vi "Processing_description.vi"(7 "type":enum16{"int", "float"}(ring)=enum."float", 8 "error in":errorcluster, 11 "Ответ устройства":string) -> (0 "error out":errorcluster, 2 "Param":T1, 4 "Тип/версия устройства":string, 6 "appended array":string[](array[string]))   [LabVIEW 2017, in "LV_Unicorn.lvlib"]
uses:
  LV_Unicorn.lvlib
  Control/unicorn_DescriptParam.ctl
panel:
  out "length":i32
  out "substring before match":string
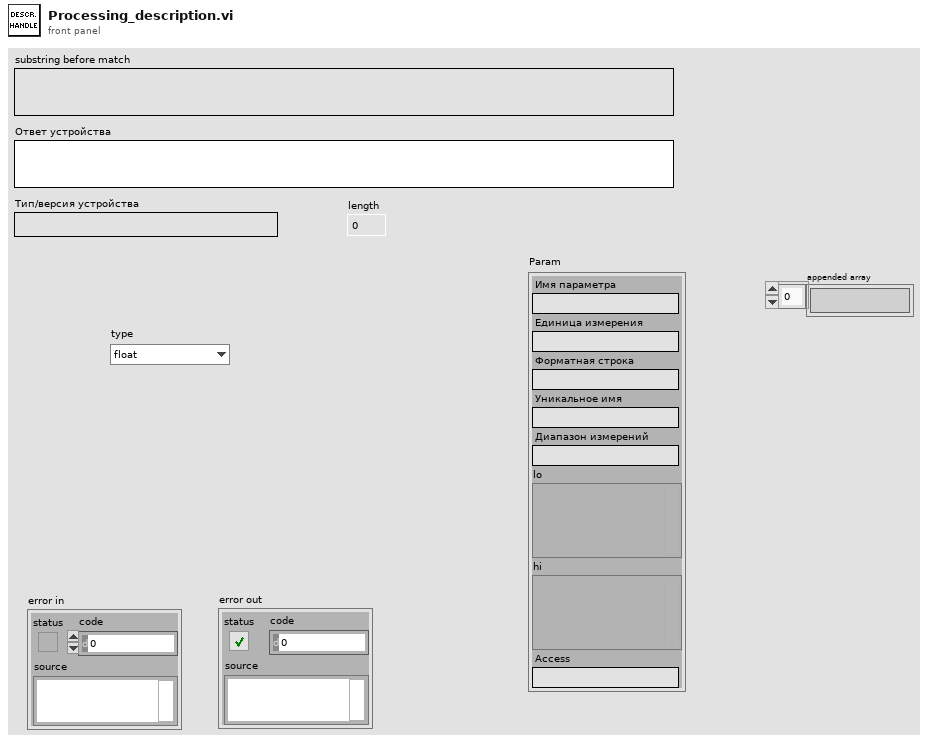
[diagram p1: front panel]
types:
  T1 = typedef "unicorn_DescriptParam.ctl" = cluster{"Имя параметра":string, "Единица измерения":string, "Форматная строка ":string, "Уникальное имя":string, "Диапазон измерений":string, "lo":variant, "hi":variant, "Access":string}
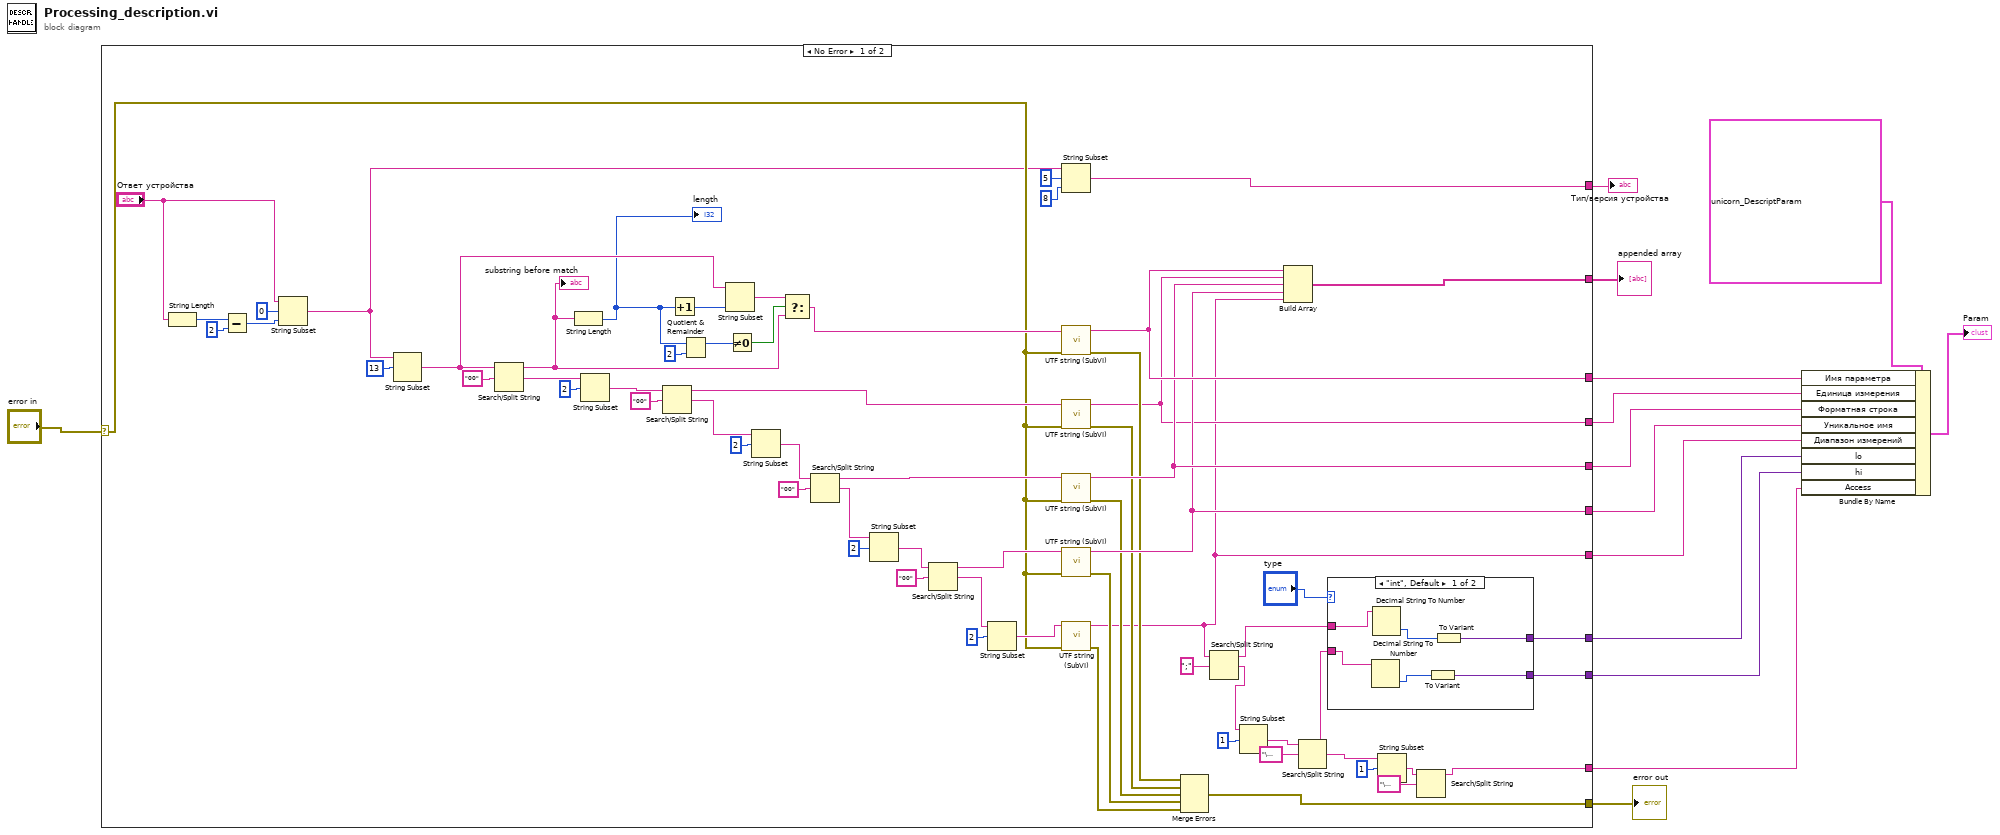
[diagram p0: block diagram]
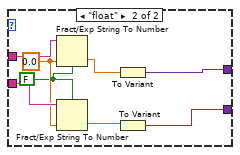
[diagram p2: hidden frame]
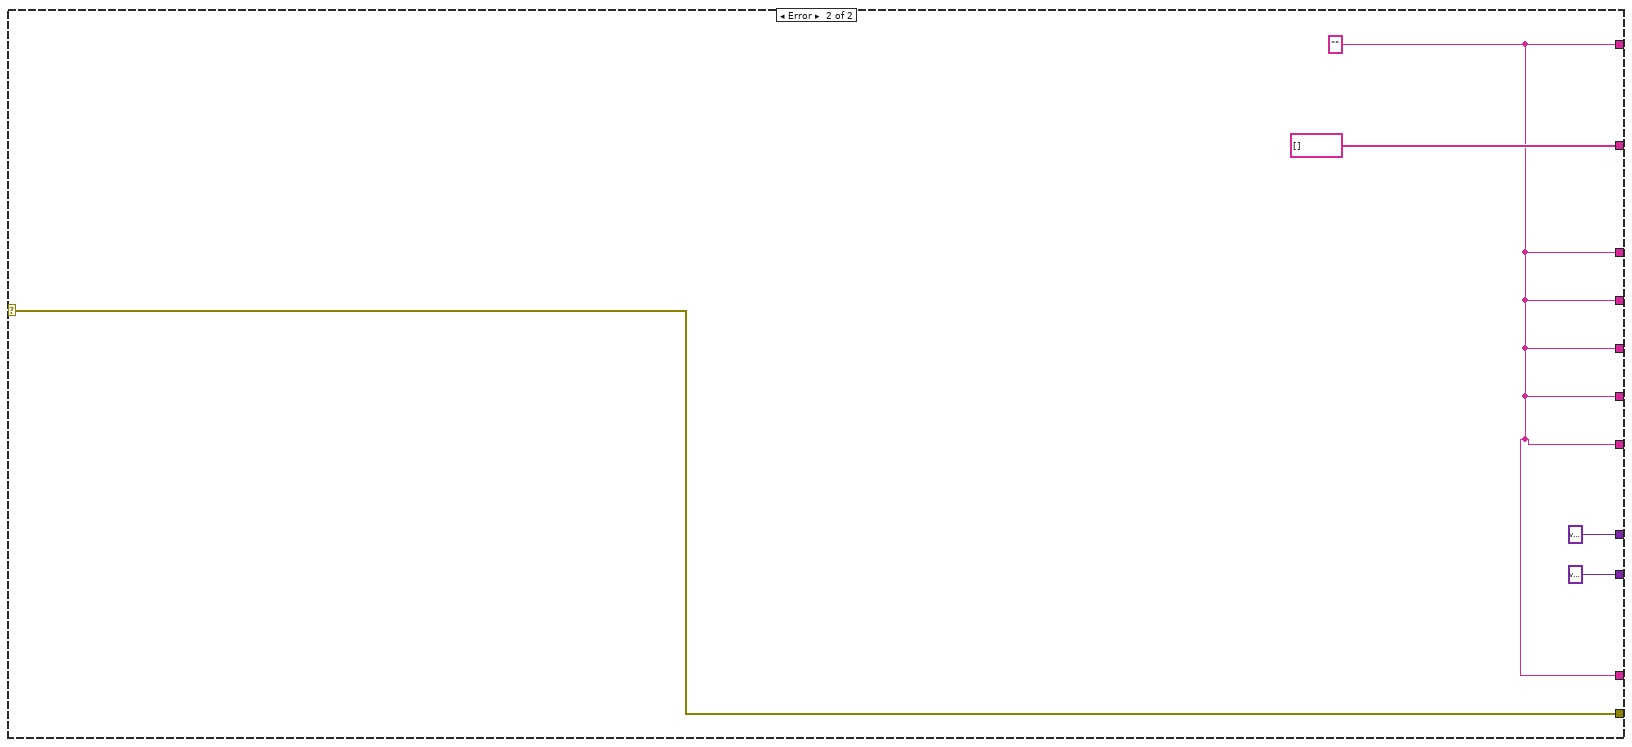
[diagram p3: hidden frame]
diagram:
  n1 = case shown="No Error" "error in" {
    selector: "error in" -> [w34 w98]
    tunnel: [w55 w95] -> w14
    tunnel: [w44 w95] -> w9
    tunnel: [w30 w95] -> w8
    tunnel: [w43 w95] -> w7
    tunnel: [w42 w95] -> w6
    tunnel: [w41 string[] []] -> w13
    tunnel: [w29 w95] -> w5
    tunnel: [w35 w98] -> w12
    tunnel: [w28 variant ("Variant")] -> w4
    tunnel: [w27 variant ("Variant")] -> w3
    tunnel: [w18 w95] -> w2
    frame No Error {
      n2 = String Length(string="Ответ устройства") -> (length=w60:i32)
      n3 = Subtract(x=w60, y=2) -> (x-y=w57:i32)
      n4 = String Subset(string="Ответ устройства", offset (0)=0 ("length (rest)"), length (rest)=w57) -> (substring=w31:string)
      n5 = String Subset(string=w31, offset (0)=13) -> (substring=w50:string)  [unwired: 1 in]
      n6 = Search/Split String(string=w50, search string/char (-)="00") -> (substring before match=w46:string, match + rest of string=w78:string)  [unwired: 1 in, 1 out]
      "substring before match" <- w46
      n7 = String Length(string=w46) -> (length=w49:i32)
      "length" <- w49
      n8 = String Subset(string=w78, offset (0)=2) -> (substring=w76:string)  [unwired: 1 in]
      n9 = Search/Split String(string=w76, search string/char (-)="00") -> (substring before match=w72:string, match + rest of string=w73:string)  [unwired: 1 in, 1 out]
      n10 = Increment(x=w49) -> (x+1=w48:i32)
      n11 = Quotient & Remainder(x=w49, y=2) -> (x-y*floor(x/y)=w52:i32)  [unwired: 1 out]
      n12 = String Subset(string=w50, length (rest)=w48) -> (substring=w47:string)  [unwired: 1 in]
      n13 = Not Equal To 0?(x=w52) -> (x != 0?=w51:bool)
      n14 = String Subset(string=w73, offset (0)=2) -> (substring=w71:string)  [unwired: 1 in]
      n15 = Select(t=w47, s=w51, f=w46) -> (s? t:f=w45:string)
      n16 = Search/Split String(string=w71, search string/char (-)="00") -> (substring before match=w69:string, match + rest of string=w67:string)  [unwired: 1 in, 1 out]
      n17 = String Subset(string=w67, offset (0)=2) -> (substring=w66:string)  [unwired: 1 in]
      n18 = Search/Split String(string=w66, search string/char (-)="00") -> (substring before match=w64:string, match + rest of string=w62:string)  [unwired: 1 in, 1 out]
      n19 = String Subset(string=w62, offset (0)=2) -> (substring=w61:string)  [unwired: 1 in]
      n20 = String Subset(string=w31, offset (0)=5, length (rest)=8 ("length (rest)")) -> (substring=w55:string)
      n21 = call "UTF string (SubVI).vi"("error in"=w34, "StringIn"=w45) -> ("error out"=w40:errorcluster, "StringOut"=w44:string)  [unwired: 8 in]
      n22 = call "UTF string (SubVI).vi"("error in"=w34, "StringIn"=w72) -> ("error out"=w39:errorcluster, "StringOut"=w30:string)  [unwired: 8 in]
      n23 = call "UTF string (SubVI).vi"("error in"=w34, "StringIn"=w69) -> ("error out"=w38:errorcluster, "StringOut"=w43:string)  [unwired: 8 in]
      n24 = call "UTF string (SubVI).vi"("error in"=w34, "StringIn"=w64) -> ("error out"=w37:errorcluster, "StringOut"=w42:string)  [unwired: 8 in]
      n25 = call "UTF string (SubVI).vi"("error in"=w34, "StringIn"=w61) -> ("error out"=w36:errorcluster, "StringOut"=w29:string)  [unwired: 8 in]
      n26 = Merge Errors(w40, w39, w38, w37, w36) -> (w35:errorcluster)
      n27 = Search/Split String(string=w29, search string/char (-)=";") -> (substring before match=w24:string, match + rest of string=w25:string)  [unwired: 1 in, 1 out]
      n28 = String Subset(string=w25, offset (0)=1) -> (substring=w17:string)  [unwired: 1 in]
      n29 = Build Array(w44, w30, w43, w42, w29) -> (w41:string[])
      n30 = Search/Split String(string=w17, search string/char (-)="\u0000") -> (substring before match=w16:string, match + rest of string=w22:string)  [unwired: 1 in, 1 out]
      n31 = case shown="\"int\", Default" "type" {
        tunnel: w16 -> [w82 w91]
        tunnel: [w86 w94] -> w28
        tunnel: [w85 w93] -> w27
        tunnel: w24 -> [w84 w92]
        frame "int", Default {
          n32 = Decimal String To Number(string=w82) -> (number=w81:i32)  [unwired: 2 in, 1 out]
          n33 = Decimal String To Number(string=w84) -> (number=w83:i32)  [unwired: 2 in, 1 out]
          n34 = To Variant(anything=w81) -> (Variant=w85:variant)
          n35 = To Variant(anything=w83) -> (Variant=w86:variant)
        }
        frame "float" {
          w87 = FALSE ("use system decimal point (T)")
          w90 = sgl 0.0 ("default (0 DBL)")
          n36 = Fract/Exp String To Number(use system decimal point (T)=w87, string=w92, default (0 dbl)=w90) -> (number=w89:sgl)  [unwired: 1 in, 1 out]
          n37 = Fract/Exp String To Number(use system decimal point (T)=w87, string=w91, default (0 dbl)=w90) -> (number=w88:sgl)  [unwired: 1 in, 1 out]
          n38 = To Variant(anything=w89) -> (Variant=w94:variant)
          n39 = To Variant(anything=w88) -> (Variant=w93:variant)
        }
      }
      n40 = String Subset(string=w22, offset (0)=1) -> (substring=w19:string)  [unwired: 1 in]
      n41 = Search/Split String(string=w19, search string/char (-)="\u0000") -> (substring before match=w18:string)  [unwired: 1 in, 2 out]
    }
    frame Error {
      w95 = "" ("Ответ устройства")
    }
  }
  "Тип/версия устройства" <- w14
  "appended array" <- w13
  "error out" <- w12
  n42 = Bundle By Name(cluster=T1 {"Имя параметра"="", "Единица измерения"="", "Форматная строка "="", "Уникальное имя"="", "Диапазон измерений"="", "lo"=variant, "hi"=variant, "Access"=""} ("Param"), "Имя параметра"=w9, "Единица измерения"=w8, "Форматная строка"=w7, "Уникальное имя"=w6, "Диапазон измерений"=w5, "lo"=w4, "hi"=w3, "Access"=w2) -> (→"Param":T1)
